vi "Find Project Dependencies in Given Maps.vi"(5 "Exclude Own Project Files?(T)":bool=TRUE, 7 "To Lower Case?(T)":bool=TRUE, 8 "Error In":errorcluster, 9 "External Targets":T3[](array[typedef]), 10 "Internal Targets":T2[](array[typedef]), 11 "Project Path in":path) -> (0 "Error Out":errorcluster, 1 "Found External Dependencies":T1[](array[typedef]), 2 "Found Internal Dependencies":T1[](array[typedef]), 3 "Project Path dub":path)   [LabVIEW 2019, in "Project.Dependencies Finder.lvlib"]
doc: "Parse a project file for internal and external dependencies.\n\nInternal dependencies are expected to have 'paths' like vi.lib\\ and should be found inside the LabVIEW folder.\nExternal dependencies are identified by unique folder names.\n\n2020-11-11: Henrik Dueholm Hansen"
uses:
  Project.Dependencies Finder.lvlib
  Ctl/Ctl_External Target Element.ctl
  Ctl/Ctl_Internal Target Element.ctl
  Ctl/Ctl_Dependency Element.ctl
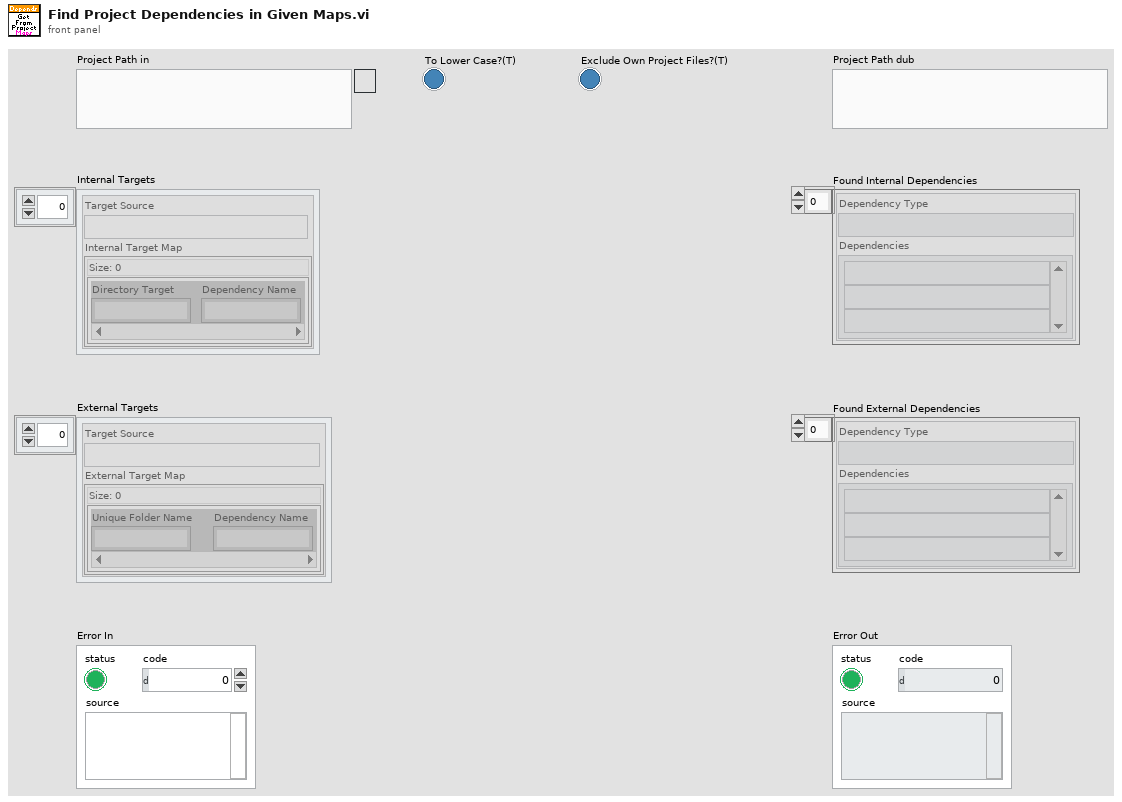
[diagram p1: front panel]
types:
  T1 = typedef "Project.Dependencies Finder.lvlib/Ctl_Dependency Element.ctl" = cluster{"Dependency Type":string, "Dependencies":string[]}
  T2 = typedef "Project.Dependencies Finder.lvlib/Ctl_Internal Target Element.ctl" = cluster{"Target Source":string, "Internal Target Map":map{string, string}}
  T3 = typedef "Project.Dependencies Finder.lvlib/Ctl_External Target Element.ctl" = cluster{"Target Source":string, "External Target Map":map{string, string}}
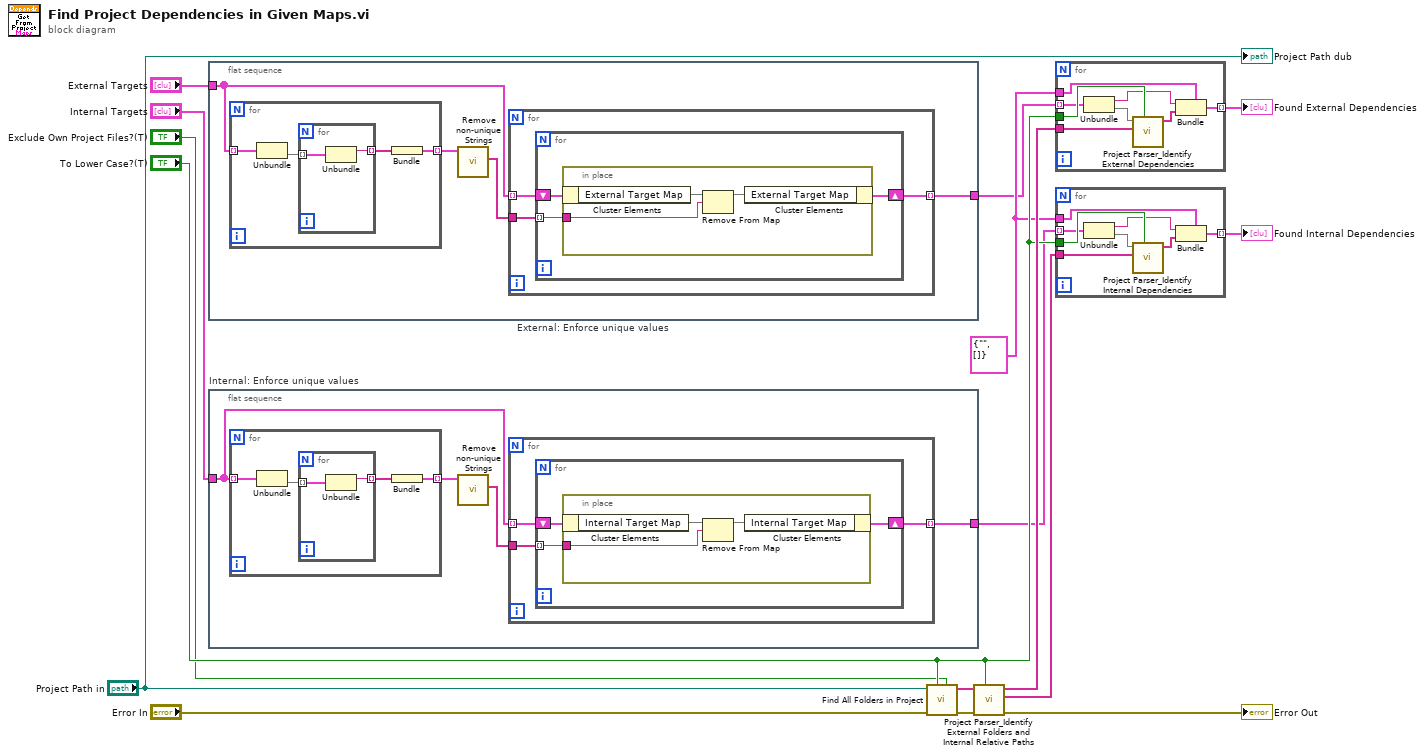
[diagram p0: block diagram]
diagram:
  w9 = T1 {"Dependency Type"="", "Dependencies"=[]} ("External Target Element")
  n1 = flat-sequence "External: Enforce unique values" {
    tunnel: "External Targets" -> [w18]
    tunnel: [w17] -> w5
    frame #0 {
      n2 = for {
        tunnel: w18 -> [w33] mode=indexing
        tunnel: [w30] -> w20 mode=indexing
        n3 = Unbundle(w33) -> ("External Target Map"=w32:map{string, string})  [unwired: 1 out]
        n4 = for {
          tunnel: w32 -> [w35] mode=indexing
          tunnel: [w34] -> w31 mode=indexing
          n5 = Unbundle(w35) -> ("Unique Folder Name"=w34:string)  [unwired: 1 out]
        }
        n6 = Bundle(w31) -> (w30:cluster{string[]})  [unwired: 1 in]
      }
      n7 = call "Remove non-unique Strings.vi"("String Array in"=w20) -> ("Removed Strings"=w19:string[])  [unwired: 9 in, 1 out]
      n8 = for {
        tunnel: w19 -> [w22]
        tunnel: w18 -> [w23] mode=indexing
        tunnel: [w21] -> w17 mode=indexing
        n9 = for {
          tunnel: w22 -> [w24] mode=indexing
          shift-right: [w25] -> w21
          shift-left: w23 -> [w26]
          n10 = in-place {
            in-place-border: w24 -> [w28]
            n11 = in-place-cluster #1(w26) -> ("External Target Map"=w29:map{string, string})
            n12 = Remove From Map(10:w28, 11:w29) -> (3:w27:map{string, string})  [unwired: 2 out]
            n13 = in-place-cluster #1("External Target Map"=w27) -> (w25:T3)
          }
        }
      }
    }
  }
  n14 = flat-sequence "Internal: Enforce unique values" {
    tunnel: "Internal Targets" -> [w37]
    tunnel: [w36] -> w3
    frame #0 {
      n15 = for {
        tunnel: w37 -> [w52] mode=indexing
        tunnel: [w49] -> w38 mode=indexing
        n16 = Unbundle(w52) -> ("Internal Target Map"=w51:map{string, string})  [unwired: 1 out]
        n17 = for {
          tunnel: w51 -> [w54] mode=indexing
          tunnel: [w53] -> w50 mode=indexing
          n18 = Unbundle(w54) -> ("Directory Target"=w53:string)  [unwired: 1 out]
        }
        n19 = Bundle(w50) -> (w49:cluster{string[]})  [unwired: 1 in]
      }
      n20 = call "Remove non-unique Strings.vi"("String Array in"=w38) -> ("Removed Strings"=w39:string[])  [unwired: 9 in, 1 out]
      n21 = for {
        tunnel: w39 -> [w40]
        tunnel: w37 -> [w42] mode=indexing
        tunnel: [w41] -> w36 mode=indexing
        n22 = for {
          tunnel: w40 -> [w43] mode=indexing
          shift-right: [w44] -> w41
          shift-left: w42 -> [w45]
          n23 = in-place {
            in-place-border: w43 -> [w47]
            n24 = in-place-cluster #2(w45) -> ("Internal Target Map"=w48:map{string, string})
            n25 = Remove From Map(10:w47, 11:w48) -> (3:w46:map{string, string})  [unwired: 2 out]
            n26 = in-place-cluster #2("Internal Target Map"=w46) -> (w44:T2)
          }
        }
      }
    }
  }
  n27 = call "Find All Folders in Project.vi"("Exclude Own Project Files?(T)"="Exclude Own Project Files?(T)", "To Lower Case?(T)"="To Lower Case?(T)", "error in (no error)"="Error In", "Project Path"="Project Path in") -> ("error out"=w14:errorcluster, "Project Folders"=w2:string[])  [unwired: 5 in, 1 out]
  n28 = call "Project Parser_Identify External Folders and Internal Relative Paths.vi"("To Lower Case?(T)"="To Lower Case?(T)", "error in (no error)"=w14, "Project Folders"=w2) -> ("error out"=→"Error Out":errorcluster, "Relateive Internals"=w11:string[], "External Combinations"=w12:string[])  [unwired: 6 in]
  n29 = for {
    tunnel: w12 -> [w62]
    tunnel: "To Lower Case?(T)" -> [w61]
    tunnel: w5 -> [w60] mode=indexing
    tunnel: w9 -> [w58]
    tunnel: [w55] -> w8 mode=indexing
    n30 = Unbundle(w60) -> ("Target Source"=w57:string, "External Target Map"=w59:map{string, string})
    n31 = call "Project Parser_Identify External Dependencies.vi"("To Lower Case?(T)"=w61, "External Folder Names"=w62, "External Target Map"=w59) -> ("Found External Dependencies"=w56:string[])  [unwired: 8 in]
    n32 = Bundle(cluster=w58, "Dependency Type"=w57, "Dependencies"=w56) -> (w55:T1)
  }
  "Found External Dependencies" <- w8
  n33 = for {
    tunnel: w11 -> [w70]
    tunnel: "To Lower Case?(T)" -> [w69]
    tunnel: w3 -> [w68] mode=indexing
    tunnel: w9 -> [w66]
    tunnel: [w63] -> w7 mode=indexing
    n34 = Unbundle(w68) -> ("Target Source"=w65:string, "Internal Target Map"=w67:map{string, string})
    n35 = call "Project Parser_Identify Internal Dependencies.vi"("To Lower Case?(T)"=w69, "Internal Relative Paths"=w70, "Internal Target Map"=w67) -> ("Found Internal Dependencies"=w64:string[])  [unwired: 8 in]
    n36 = Bundle(cluster=w66, "Dependency Type"=w65, "Dependencies"=w64) -> (w63:T1)
  }
  "Found Internal Dependencies" <- w7
  "Project Path dub" <- "Project Path in"
